vi "FPGA_DIOWritePWMPeriod.vi"(10 "PWMPeriod":u16=1509, 11 "DIODeviceRef In":T1) -> (3 "DIODeviceRef Out":T1)   [LabVIEW 2017]
uses:
  <vilib>/Rock Robotics/SystemInterfaces/DIO/FPGA_DIODevRef.ctl
  <vilib>/Rock Robotics/SystemInterfaces/System/FPGA_SystemFPGA Ref Global.vi
  <vilib>/Utility/error.llb/Error Cluster From Error Code.vi
  <vilib>/rvi/errors/niLvFpgaAdjustHostInterfaceError.vi
  <vilib>/rvi/interface/nirviReadWriteControl/nirviReadWriteControl.xnode
  <vilib>/Rock Robotics/SystemInterfaces/System/FPGA_SystemFRC FPGA Ref.ctl
  <vilib>/rvi/interface/Simulation/niFpgaSimulationCallBeginRW.vi
  NiFpgaLv.dll
panel:
  out "error out":errorcluster
  in  "error in (no error)":errorcluster
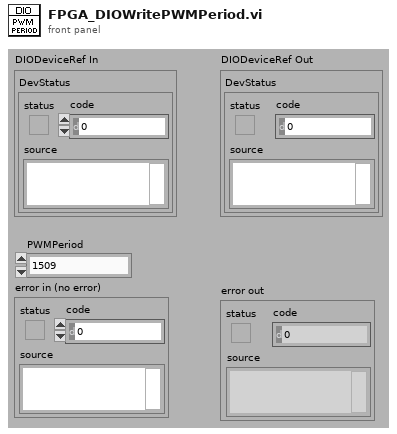
[diagram p1: front panel]
types:
  T1 = typedef "FPGA_DIODevRef.ctl" = cluster{"DevStatus":errorcluster}
  T2 = typedef "FPGA_SystemFRC FPGA Ref.ctl" = refnum<k20>
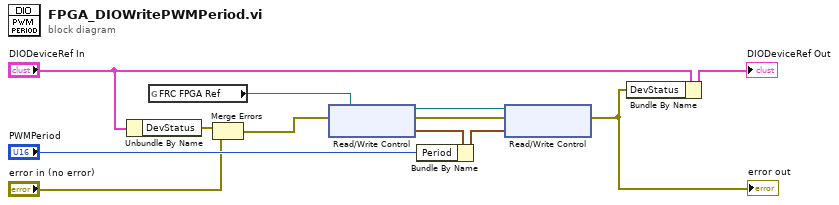
[diagram p0: block diagram]
diagram:
  n1 = Unbundle By Name("DIODeviceRef In") -> ("DevStatus"=w10:errorcluster)
  n2 = global read "FPGA_SystemFPGA Ref Global.vi" "FRC FPGA Ref"() -> (w2:T2)
  n3 = Merge Errors(w10, "error in (no error)") -> (w9:errorcluster)
  n4 = xnode "Read/Write Control"("FPGA VI Reference In"=w2, "error in"=w9) -> ("FPGA VI Reference Out"=w6:T2, "error out"=w5:errorcluster, "PWM.Config"=w4:cluster{"Period":u16, "MinHigh":u16})
  n5 = Bundle By Name(cluster=w4, "Period"="PWMPeriod") -> (w7:cluster{"Period":u16, "MinHigh":u16})
  n6 = xnode "Read/Write Control"("FPGA VI Reference In"=w6, "error in"=w5, "PWM.Config"=w7) -> ("error out"=w11:errorcluster)  [unwired: 1 out]
  "error out" <- w11
  n7 = Bundle By Name(cluster="DIODeviceRef In", "DevStatus"=w11) -> (→"DIODeviceRef Out":T1)
